vi "Set PID.vi"(5 "Output #":i32=1, 6 "D":dbl, 7 "P manual":dbl, 8 "error in (no error)":errorcluster, 9 "I":dbl, 10 "P":dbl, 11 "Temperature Controller in":refnum<class "Temperature Controller.lvclass">) -> (0 "error out":errorcluster, 3 "Temperature Controller out":refnum<class "Temperature Controller.lvclass">)   [LabVIEW 2021, in "Temperature Controller.lvclass"]
uses:
  Temperature Controller.lvclass
  Read T ctl driver.vi
  Write T ctl driver.vi
  NHMFL_Core/Libraries/Instruments/Temperature Controller Driver/Temperature Controller Driver.lvclass
  Temperature Controller.lvclass/Temperature Controller.ctl
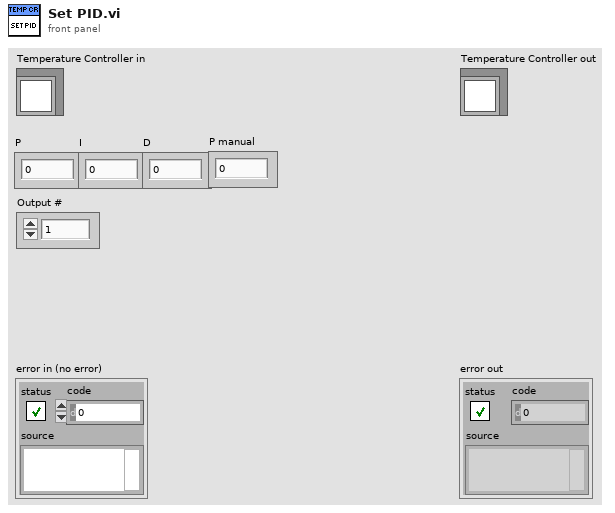
[diagram p1: front panel]
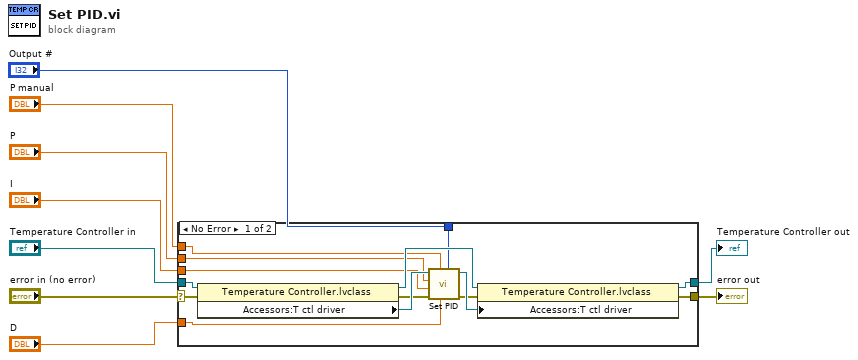
[diagram p0: block diagram]
diagram:
  n1 = case shown="No Error" "error in (no error)" {
    selector: "error in (no error)" -> [w23 w25]
    tunnel: [w17 w25] -> w8
    tunnel: [w16 w24] -> w6
    tunnel: "Temperature Controller in" -> [w22 w24]
    tunnel: "P manual" -> [w14 _]
    tunnel: "P" -> [w13 _]
    tunnel: "I" -> [w12 _]
    tunnel: "D" -> [w11 _]
    tunnel: "Output #" -> [w10 _]
    frame No Error {
      n2 = property class="Temperature Controller.lvclass"(reference=w22, error in=w23) -> (reference out=w15:refnum<class "Temperature Controller.lvclass">, error out=w20:errorcluster, "Accessors:T ctl driver"=w21:refnum<class "Temperature Controller Driver.lvclass">)
      n3 = call-dynamic "Set PID.vi"("Output #"=w10, "D"=w11, "P manual"=w14, "error in (no error)"=w20, "I"=w12, "P"=w13, "Temperature Controller Driver in"=w21) -> ("error out"=w18:errorcluster, "Temperature Controller Driver out"=w19:refnum<class "Temperature Controller Driver.lvclass">)  [unwired: 3 in]
      n4 = property class="Temperature Controller.lvclass"(reference=w15, error in=w18, "Accessors:T ctl driver"=w19) -> (reference out=w16:refnum<class "Temperature Controller.lvclass">, error out=w17:errorcluster)
    }
    frame Error {
    }
  }
  "error out" <- w8
  "Temperature Controller out" <- w6
